vi "LIDAR Stop.vi"() -> ()   [LabVIEW 2016]
panel:
  in  "LIDAR Stop":bool
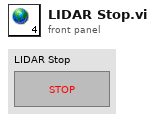
[diagram p1: front panel]
diagram:
